vi "PPL_DRIVE_Set_Wheel_Dist.vi"(9 "Right Wheel Dist M":dbl format="%17.2f", 11 "Left Wheel Dist M":dbl format="%17.2f") -> ()   [LabVIEW 2019]
uses:
  PPL_DRIVE_GLOBALS.vi
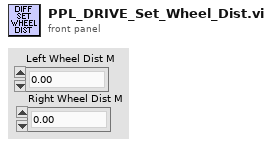
[diagram p1: front panel]
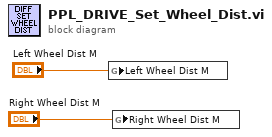
[diagram p0: block diagram]
diagram:
  n1 = global write "PPL_DRIVE_GLOBALS.vi" "Left Wheel Dist M"("Left Wheel Dist M") -> ()
  n2 = global write "PPL_DRIVE_GLOBALS.vi" "Right Wheel Dist M"("Right Wheel Dist M") -> ()
